vi "Meas Proc QWTB Generate Algorithm Info Section.vi"(7 "processing setup":T1={"mode"=enum."Raw", "call after avgs?"=FALSE, "calculate?"=FALSE, "raw mode"={"command"="", "result mode"=enum."Display console output (only Octave)", "res variable"=""}, "QWTB"={"QWTB path"=path "", "alg filter path"="", "alg ids"=[], "alg parameters"=[], "parsed parameters"=[], "selected alg id"="", "selected unc mode"=enum."None", "qwtb mcc"=100, "qwtb timeout"=90, "qwtb covg"=95.0, "qwtb ofs"=0, "qwtb lim data"=0, "multicore"={"jobs folder"=path "", "cores"=0, "max jobs"=0, "mode"=enum."Singlecore"}, "unc once?"=FALSE}}, 8 "sections in":string[](array[string]), 10 "sequence item":T10, 11 "new info data in":string) -> (0 "sections out":string[](array[string]), 3 "new info data out":string)   [LabVIEW 2013]
doc: "This VI will write QWTB calculation data into the measurement info header."
uses:
  Meas Sequence Item.ctl
  Meas Sampling Configuration.ctl
  adc/ADC Trig Config.ctl
  adc/ADC Trig Mode Source.ctl
  adc/ADC Trig Coupling.ctl
  adc/ADC Trig Slope.ctl
  Meas Proc QWTB Algorithm Parameter Data.ctl
  Meas Process Config.ctl
  Meas Process Mode.ctl
  Meas Process Raw Config.ctl
  Meas Process Raw Result Mode.ctl
  Meas Proc QWTB Setup.ctl
  Meas Proc QWTB Uncertainty Mode.ctl
  Meas Proc QWTB Multicore Setup.ctl
  Meas Proc QWTB Multicore Type.ctl
  octave/infolib.lvlibp/Private/Add key polymorph parts/String.vi
  octave/infolib.lvlibp/Private/Add key polymorph parts/Boolean.vi
  octave/infolib.lvlibp/Private/Add key polymorph parts/EXT.vi
  octave/infolib.lvlibp/Private/Add matrix polymorph parts/1D String.vi
  octave/infolib.lvlibp/Private/Add key polymorph parts/I64.vi
  octave/infolib.lvlibp
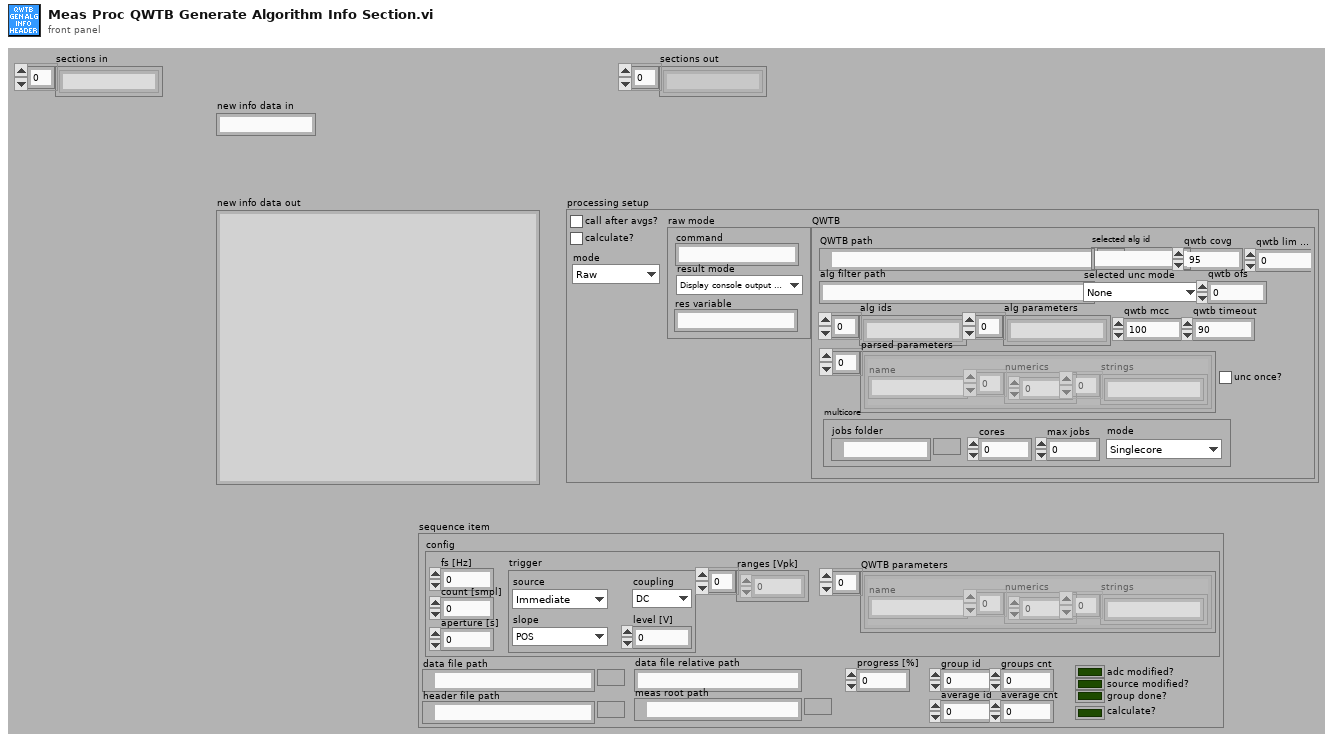
[diagram p1: front panel]
types:
  T1 = typedef "Meas Process Config.ctl" = cluster{"mode":T2, "call after avgs?":bool, "calculate?":bool, "raw mode":T3, "QWTB":T5}
  T2 = typedef "Meas Process Mode.ctl" = enum16{"Raw", "QWTB"}
  T3 = typedef "Meas Process Raw Config.ctl" = cluster{"command":string, "result mode":T4, "res variable":string}
  T4 = typedef "Meas Process Raw Result Mode.ctl" = enum16{"Display console output (only Octave)", "Display string variable", "Display result file %respath%"}
  T5 = typedef "Meas Proc QWTB Setup.ctl" = cluster{"QWTB path":path, "alg filter path":string, "alg ids":string[], "alg parameters":string[], "parsed parameters":T6[], "selected alg id":string, "selected unc mode":T7, "qwtb mcc":i32, "qwtb timeout":i32, "qwtb covg":dbl, "qwtb ofs":i64, "qwtb lim data":i64, "multicore":T8, "unc once?":bool}
  T6 = typedef "Meas Proc QWTB Algorithm Parameter Data.ctl" = cluster{"name":string, "numerics":dbl[], "strings":string[]}
  T7 = typedef "Meas Proc QWTB Uncertainty Mode.ctl" = enum16{"None", "GUF", "Monte Carlo"}
  T8 = typedef "Meas Proc QWTB Multicore Setup.ctl" = cluster{"jobs folder":path, "cores":i32, "max jobs":i32, "mode":T9}
  T9 = typedef "Meas Proc QWTB Multicore Type.ctl" = enum16{"Singlecore", "Multicore", "Multistation"}
  T10 = typedef "Meas Sequence Item.ctl" = cluster{"config":T11, "data file path":path, "header file path":path, "group id":i32, "average id":i32, "group done?":bool, "adc modified?":bool, "source modified?":bool, "progress [%]":dbl, "groups cnt":i32, "average cnt":i32, "data file relative path":string, "meas root path":path, "calculate?":bool}
  T11 = typedef "Meas Sampling Configuration.ctl" = cluster{"fs [Hz]":dbl, "count [smpl]":i64, "aperture [s]":dbl, "trigger":T12, "ranges [Vpk]":dbl[], "QWTB parameters":T6[]}
  T12 = typedef "ADC Trig Config.ctl" = cluster{"source":T13, "level [V]":dbl, "coupling":T14, "slope":T15}
  T13 = typedef "ADC Trig Mode Source.ctl" = enum16{"Immediate", "External", "Level"}
  T14 = typedef "ADC Trig Coupling.ctl" = enum16{"DC", "AC"}
  T15 = typedef "ADC Trig Slope.ctl" = enum16{"POS", "NEG"}
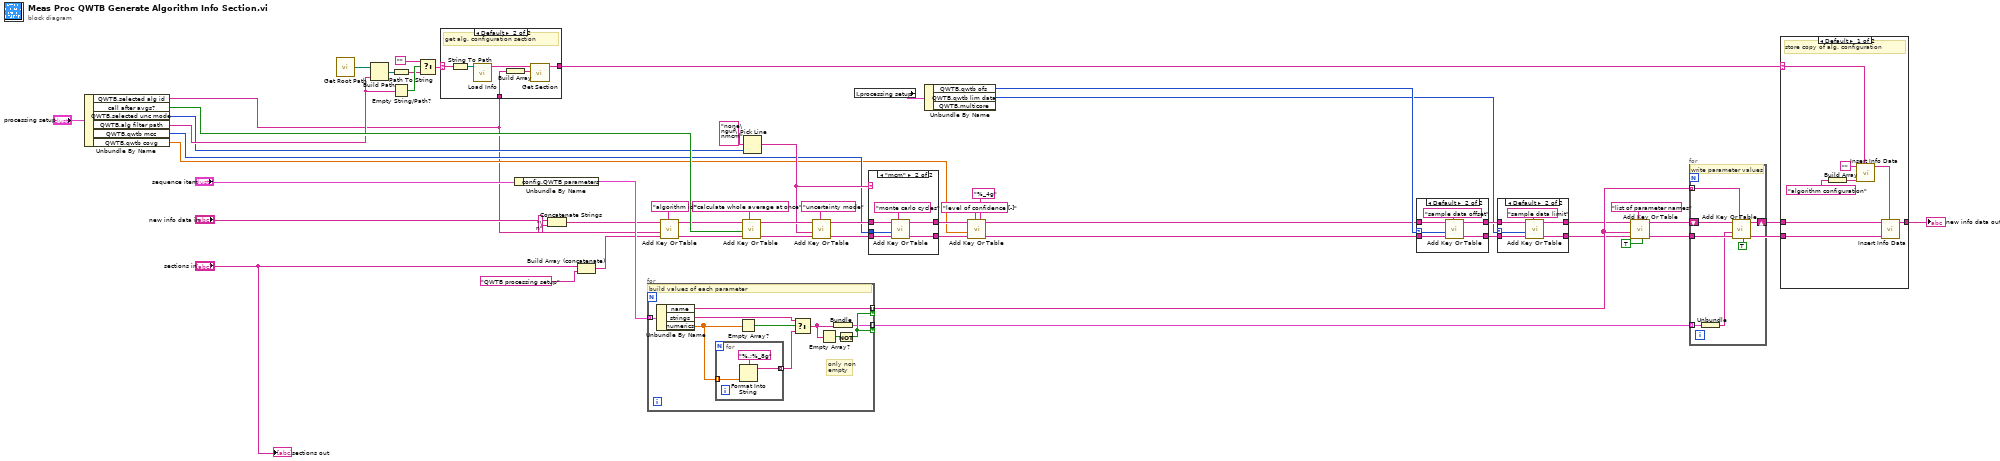
[diagram p0: block diagram]
diagram:
  n1 = Unbundle By Name("processing setup") -> ("QWTB.selected alg id"=w10:string, "call after avgs?"=w50:bool, "QWTB.selected unc mode"=w21:T7, "QWTB.alg filter path"=w49:string, "QWTB.qwtb mcc"=w16:i32, "QWTB.qwtb covg"=w12:dbl)
  n2 = call "Get Root Path.vi"() -> ("root path"=w23:path)
  n3 = Build Path(base path=w23, name or relative path=w49) -> (appended path=w35:path)
  n4 = Path To String(path=w35) -> (string=w24:string)
  n5 = Empty String/Path?(string/path=w49) -> (empty?=w34:bool)
  n6 = Select(t="", s=w34, f=w24) -> (s? t:f=w25:string)
  n7 = case shown="Default" w25 {
    selector: w25 -> [_ w60]
    tunnel: w10 -> [_ w58]
    tunnel: [_ w56] -> w26
    frame "" {
    }
    frame Default {
      # "get alg. configuration section"
      n8 = String To Path(string=w60) -> (path=w59:path)
      n9 = call "Load Info.vi"("filename"=w59) -> ("info data"=w55:string)  [unwired: 9 in, 1 out]
      n10 = Build Array(w58) -> (w57:string[])
      n11 = call "Get Section.vi"("sections"=w57, "info data"=w55) -> ("section part"=w56:string)  [unwired: 8 in, 1 out]
    }
  }
  n12 = Unbundle By Name("sequence item") -> ("config.QWTB parameters"=w45:T6[])
  n13 = Concatenate Strings("new info data in", "\n" ("string")) -> (w39:string)
  n14 = Build Array (concatenate)("sections in", "QWTB processing setup" ("section name")) -> (w40:string[])
  n15 = for {
    tunnel: w45 -> [w70] mode=indexing
    tunnel: [w69] -> w28 mode=indexing if=w63
    tunnel: [w61] -> w30 mode=indexing if=w63
    # "only non\nempty"
    # "build values of each parameter"
    n16 = Unbundle By Name(w70) -> ("name"=w69:string, "strings"=w66:string[], "numerics"=w68:dbl[])
    n17 = for {
      tunnel: w68 -> [w72] mode=indexing
      tunnel: [w71] -> w65 mode=indexing
      n18 = Format Into String(format string="%.;%_8g", w72) -> (resulting string=w71:string)  [unwired: 2 in, 1 out]
    }
    n19 = Empty Array?(array=w68) -> (empty?=w67:bool)
    n20 = Select(t=w66, s=w67, f=w65) -> (s? t:f=w62:string[])
    n21 = Empty Array?(array=w62) -> (empty?=w64:bool)
    n22 = Bundle("strings"=w62) -> (w61:cluster{"strings":string[]})  [unwired: 1 in]
    n23 = Not(x=w64) -> (.not. x?=w63:bool)
  }
  n24 = call-poly "Add Key Or Table.vi"("key description"="algorithm id", "sections"=w40, "string"=w10, "info data"=w39) -> ("sections out"=w42:string[], "info data out"=w41:string)  [unwired: 6 in]
  n25 = call-poly "Add Key Or Table.vi"("key description"="calculate whole average at once", "sections"=w42, "boolean"=w50, "info data"=w41) -> ("sections out"=w38:string[], "info data out"=w37:string)  [unwired: 6 in]
  n26 = Pick Line(multi-line string="none\nguf\nmcm", line index=w21) -> (output string=w17:string)  [unwired: 1 in]
  n27 = call-poly "Add Key Or Table.vi"("key description"="uncertainty mode", "sections"=w38, "string"=w17, "info data"=w37) -> ("sections out"=w18:string[], "info data out"=w19:string)  [unwired: 6 in]
  n28 = local read "processing setup"() -> (w9:T1)
  n29 = case shown="\"mcm\"" w17 {
    tunnel: w19 -> [w74 w81]
    tunnel: w18 -> [w75 w80]
    tunnel: [w75 w78] -> w13
    tunnel: [w74 w77] -> w14
    tunnel: w16 -> [_ w76]
    frame "False", Default {
    }
    frame "mcm" {
      n30 = call-poly "Add Key Or Table.vi"("key description"="monte carlo cycles", "sections"=w80, "numeric"=w76, "info data"=w81) -> ("sections out"=w78:string[], "info data out"=w77:string)  [unwired: 6 in]
    }
  }
  n31 = Unbundle By Name(w9) -> ("QWTB.qwtb ofs"=w8:i64, "QWTB.qwtb lim data"=w5:i64)  [unwired: 1 out]
  n32 = call-poly "Add Key Or Table.vi"("format string (%_20f)"="%_4g", "key description"="level of confidence [-]", "sections"=w13, "numeric"=w12, "info data"=w14) -> ("sections out"=w2:string[], "info data out"=w1:string)  [unwired: 5 in]
  n33 = case shown="Default" w8 {
    selector: w8 -> [_ w87]
    tunnel: w2 -> [w83 w89]
    tunnel: w1 -> [w82 w88]
    tunnel: [w83 w85] -> w7
    tunnel: [w82 w84] -> w6
    frame 0 {
    }
    frame Default {
      n34 = call-poly "Add Key Or Table.vi"("key description"="sample data offset", "sections"=w89, "numeric"=w87, "info data"=w88) -> ("sections out"=w85:string[], "info data out"=w84:string)  [unwired: 6 in]
    }
  }
  n35 = case shown="Default" w5 {
    selector: w5 -> [_ w95]
    tunnel: w7 -> [w91 w97]
    tunnel: w6 -> [w90 w96]
    tunnel: [w91 w93] -> w4
    tunnel: [w90 w92] -> w3
    frame 0 {
    }
    frame Default {
      n36 = call-poly "Add Key Or Table.vi"("key description"="sample data limit", "sections"=w97, "numeric"=w95, "info data"=w96) -> ("sections out"=w93:string[], "info data out"=w92:string)  [unwired: 6 in]
    }
  }
  n37 = call-poly "Add Key Or Table.vi"("column vector (F)"=TRUE, "key description"="list of parameter names", "sections"=w4, "string"=w28, "info data"=w3) -> ("sections out"=w31:string[], "info data out"=w29:string)  [unwired: 5 in]
  n38 = for {
    tunnel: w28 -> [w104] mode=indexing
    tunnel: w30 -> [w102] mode=indexing
    tunnel: w31 -> [w103]
    shift-right: [w100] -> w27
    shift-left: w29 -> [w99]
    # "write parameter values"
    n39 = Unbundle(w102) -> ("strings"=w101:string[])
    n40 = call-poly "Add Key Or Table.vi"("column vector (F)"=TRUE, "key description"=w104, "sections"=w103, "string"=w101, "info data"=w99) -> ("info data out"=w100:string)  [unwired: 5 in, 1 out]
  }
  n41 = case shown="Default" w26 {
    selector: w26 -> [w109 _]
    tunnel: w31 -> [w108 _]
    tunnel: w27 -> [w105 w113]
    tunnel: [w112 w113] -> w54
    frame Default {
      # "store copy of alg. configuration"
      n42 = Build Array("algorithm configuration" ("section name")) -> (w110:string[])
      n43 = call "Insert Info Data.vi"("info data to insert"=w109, "sections"=w110, "info data"="") -> ("info data out"=w106:string)  [unwired: 7 in, 1 out]
      n44 = call "Insert Info Data.vi"("info data to insert"=w106, "sections"=w108, "info data"=w105) -> ("info data out"=w112:string)  [unwired: 7 in, 1 out]
    }
    frame "" {
    }
  }
  "new info data out" <- w54
  "sections out" <- "sections in"
